vi "OPTICAL BEACON TRACKER.vi"() -> ()   [LabVIEW 2015]
uses:
  <vilib>/userdefined/High Color/IMAQdx.ctl
  <vilib>/vision/driver/NI_Vision_Acquisition_Software.lvlib
  <resource>/objmgr/imaqdx.rc
panel:
  out "Numeric":dbl
  out "Compared":sgl
  out "Optical Beacon Aligned":bool
  in  "Threshhold x":dbl format="%#_13g"
  in  "stop":bool
  out "GREEN X":sgl
  out "RED X":sgl
  in  "Camera":T1
  in  "Stop 3":bool
  out "VA RED IMAGE":T2(plugin-control)
  out "FEED RED":T2(plugin-control)
  out "Processed Image RED":T2(plugin-control)
  out "Video Modes":string
  in  "Video Mode":dbl min=0.0 max=5.0 step=1.0
  out "Y Resoloution":i32
  out "X Resoloution":i32
  in  "Stop 2":bool
  out "VA GREEN Image":T2(plugin-control)
  out "FEED GREEN":T2(plugin-control)
  out "Process Image GREEN":T2(plugin-control)
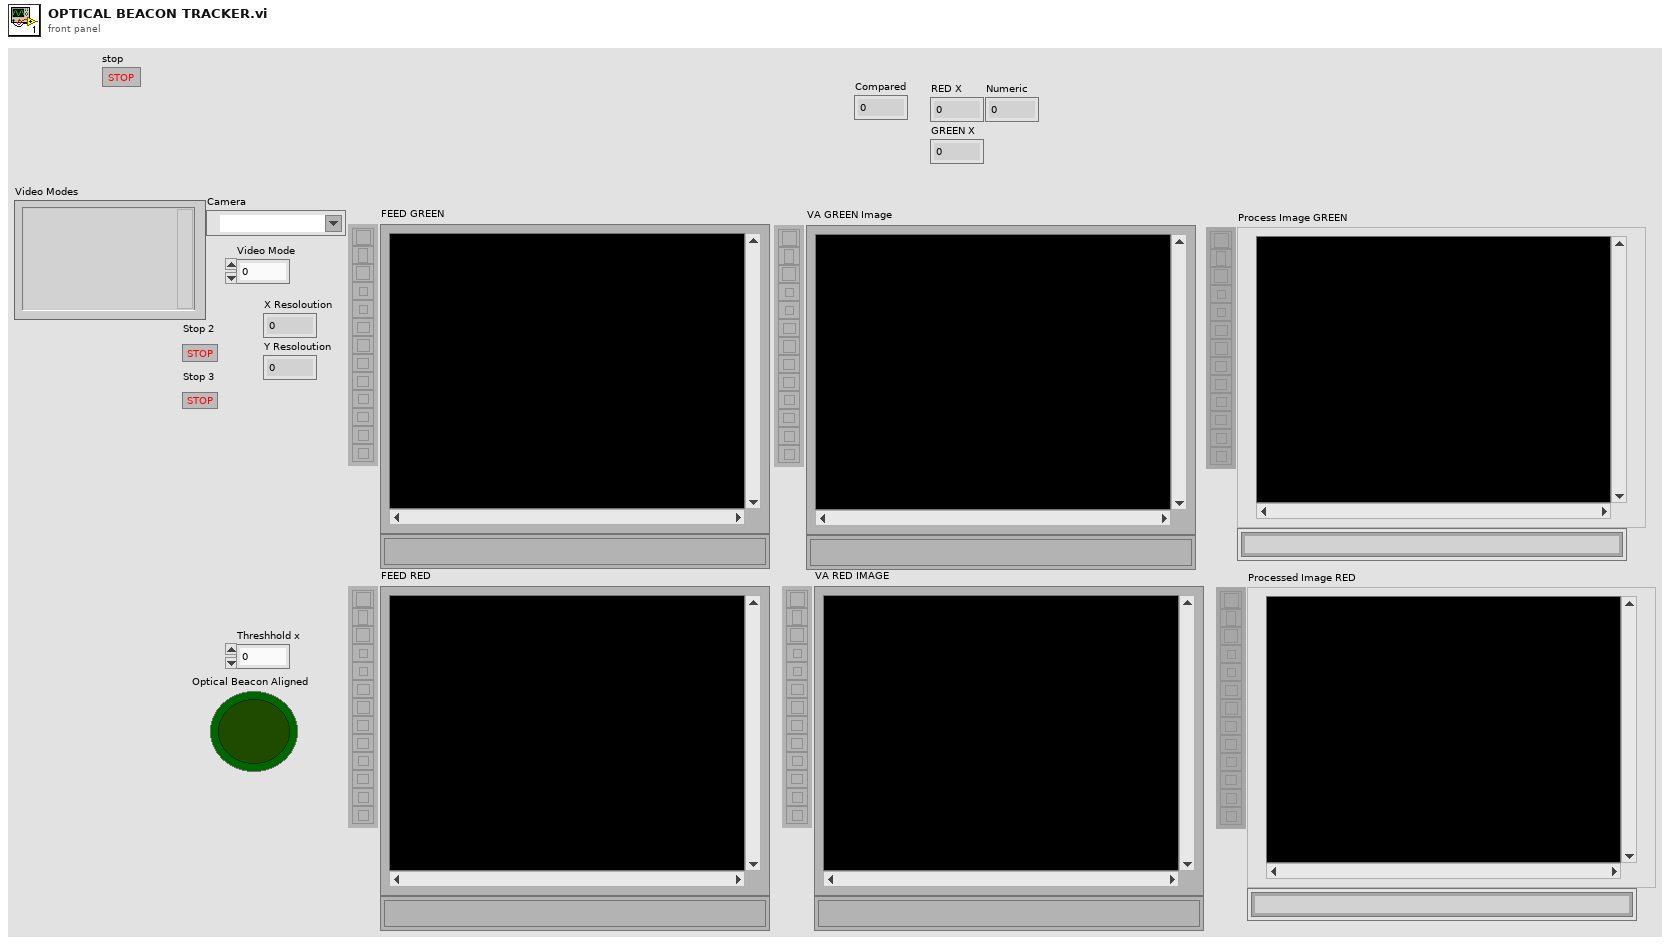
[diagram p1: front panel]
types:
  T1 = typedef "IMAQdx.ctl" = refnum<k21>
  T2 = typedef "IMAQ Image.ctl" = refnum<image>
  T3 = typedef "IMAQ Circle" = cluster{"Center X":i32, "Center Y":i32, "Inner Radius":i32, "Outer Radius":i32, "Start Angle":dbl, "End Angle":dbl}
  T4 = cluster{"Center":cluster{"X":sgl, "Y":sgl}, "Radius":dbl}
  T5 = typedef "ROI Descriptor" = cluster{"Global Rectangle":i32[], "Contours":cluster{"ID":enum32{"External", "Internal"}, "Type":u32, "Coordinates":i32[]}[]}
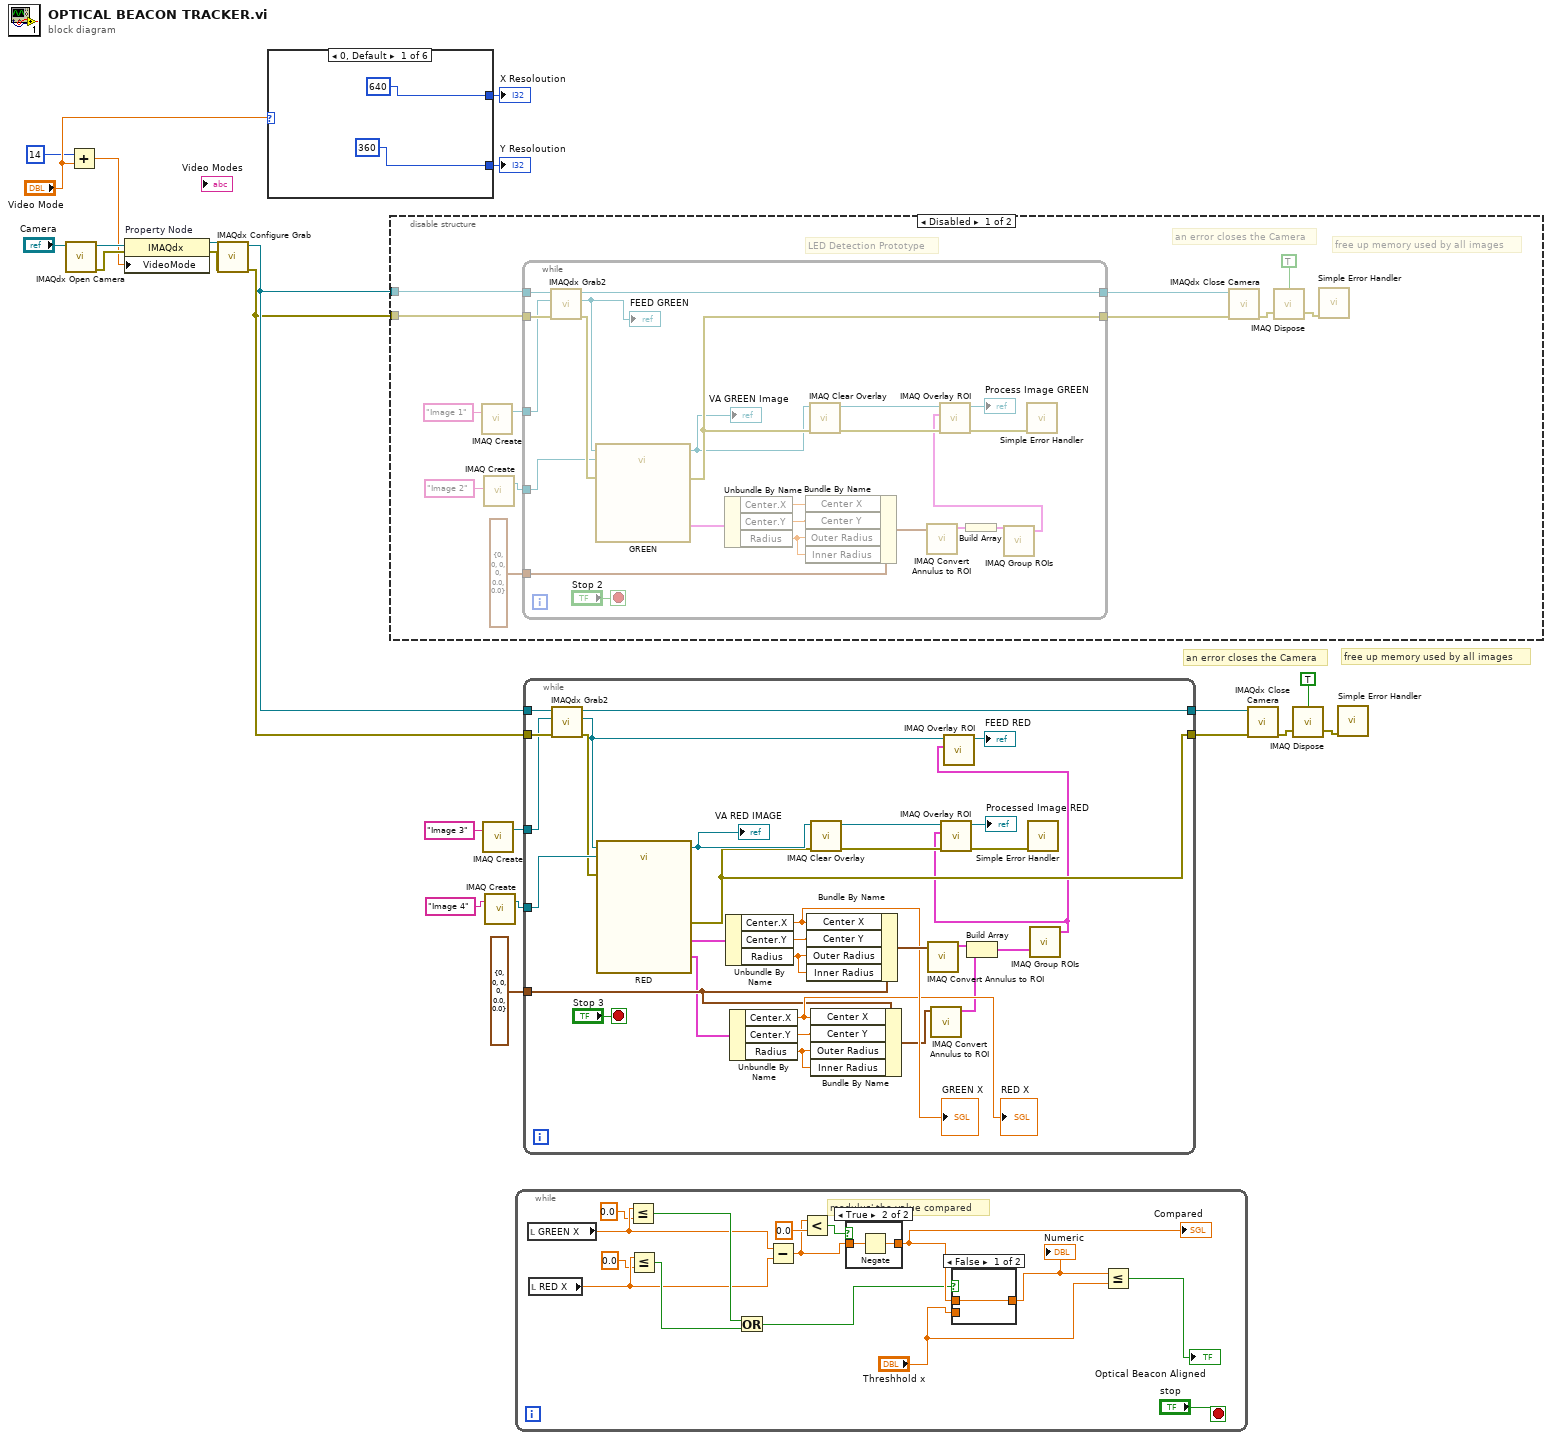
[diagram p0: block diagram]
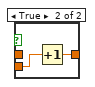
[diagram p2: hidden frame]
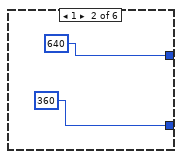
[diagram p5: hidden frame]
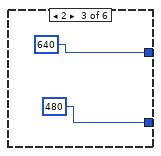
[diagram p6: hidden frame]
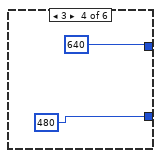
[diagram p7: hidden frame]
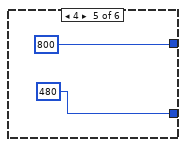
[diagram p8: hidden frame]
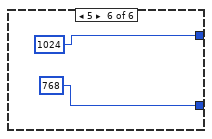
[diagram p9: hidden frame]
diagram:
  # "an error closes the Camera"
  # "free up memory used by all images"
  n1 = call <vilib>:"IMAQdx Open Camera.vi"("Session In"="Camera") -> ("error out"=w21:errorcluster, "Session Out"=w22:T1)  [unwired: 9 in]
  n2 = Add(x=14, y="Video Mode") -> (x+y=w18:dbl)
  n3 = property on="Property Node" class="IMAQdx"(reference=w22, error in=w21, "VideoMode"=w18) -> (reference out=w20:T1, error out=w19:errorcluster)
  n4 = call <vilib>:"IMAQdx Configure Grab.vi"("error in"=w19, "Session In"=w20) -> ("error out"=w4:errorcluster, "Session Out"=w5:T1)  [unwired: 8 in]
  n5 = case shown="0, Default" "Video Mode" {
    tunnel: [640 640 640 640 800 1024] -> w15
    tunnel: [360 360 480 480 480 768] -> w16
    frame 0, Default {
    }
    frame 1 {
    }
    frame 2 {
    }
    frame 3 {
    }
    frame 4 {
    }
    frame 5 {
    }
  }
  "X Resoloution" <- w15
  "Y Resoloution" <- w16
  n6 = disable-structure shown="Disabled" {
    disable-tunnel: w5 -> [w36 _]
    disable-tunnel: w4 -> [w35 _]
    frame Disabled {
      # "LED Detection Prototype"
      # "an error closes the Camera"
      # "free up memory used by all images"
      n7 = call "IMAQ Create"("Image Name"="Image 1") -> ("New Image"=w40:T2)  [unwired: 4 in, 1 out]
      n8 = call "IMAQ Create"("Image Name"="Image 2") -> ("New Image"=w43:T2)  [unwired: 4 in, 1 out]
      n9 = while {
        tunnel: [w51] -> w39
        tunnel: w43 -> [w47]
        tunnel: w35 -> [w69]
        tunnel: w36 -> [w68]
        tunnel: w40 -> [w67]
        tunnel: [w66] -> w38
        tunnel: T3 {"Center X"=0, "Center Y"=0, "Inner Radius"=0, "Outer Radius"=0, "Start Angle"=0.0, "End Angle"=0.0} ("Annulus") -> [w56]
        stop <- "Stop 2" stop-if-true
        n10 = call <vilib>:"IMAQdx Grab2.vi"("error in"=w69, "Image In"=w67, "Session In"=w68) -> ("error out"=w64:errorcluster, "Image Out"=w63:T2, "Session Out"=w66:T1)  [unwired: 5 in, 1 out]
        "FEED GREEN" <- w63
        n11 = call "GREEN"("Image In"=w63, "Image Dst"=w47, "error in"=w64) -> ("Image Out"=w49:T2, "Best Circle (Fit Circle Ball 1)"=w58:T4, "error out"=w51:errorcluster)  [unwired: 1 in, 21 out]
        "VA GREEN Image" <- w49
        n12 = Unbundle By Name(w58) -> ("Center.X"=w50:sgl, "Center.Y"=w59:sgl, "Radius"=w62:dbl)
        n13 = Bundle By Name(cluster=w56, "Center X"=w50, "Center Y"=w59, "Outer Radius"=w62, "Inner Radius"=w62) -> (w57:T3)
        n14 = call "IMAQ Clear Overlay"("error in (no error)"=w51, "Image"=w49) -> ("error out"=w54:errorcluster, "Image Out"=w53:T2)  [unwired: 1 in, 7 out]
        n15 = call "IMAQ Convert Annulus to ROI"("Annulus"=w57) -> ("ROI Descriptor"=w60:T5)  [unwired: 1 in, 8 out]
        n16 = Build Array(w60) -> (w61:T5[])
        n17 = call "IMAQ Group ROIs"("ROI Descriptors"=w61) -> ("ROI Descriptor out"=w52:T5)  [unwired: 1 in, 3 out]
        n18 = call "IMAQ Overlay ROI"("error in (no error)"=w54, "ROI Descriptor"=w52, "Image"=w53) -> ("error out"=w55:errorcluster, "Image Out"=→"Process Image GREEN":T2)  [unwired: 3 in, 4 out]
        n19 = call <vilib>:"Simple Error Handler.vi"("error in (no error)"=w55) -> ()  [unwired: 1 in, 8 out]
      }
      n20 = call <vilib>:"IMAQdx Close Camera.vi"("error in"=w39, "Session In"=w38) -> ("error out"=w44:errorcluster)  [unwired: 9 in]
      n21 = call "IMAQ Dispose"("All Images? (No)"=TRUE, "error in (no error)"=w44) -> ("error out"=w45:errorcluster)  [unwired: 4 in]
      n22 = call <vilib>:"Simple Error Handler.vi"("error in (no error)"=w45) -> ()  [unwired: 4 in, 5 out]
    }
    frame Enabled {
    }
  }
  n23 = call "IMAQ Create"("Image Name"="Image 3") -> ("New Image"=w10:T2)  [unwired: 4 in, 1 out]
  n24 = call "IMAQ Create"("Image Name"="Image 4") -> ("New Image"=w9:T2)  [unwired: 4 in, 1 out]
  n25 = while {
    stop <- "stop" stop-if-true
    # "modulus' the value compared"
    n26 = local read "GREEN X"() -> (w73:sgl)
    n27 = local read "RED X"() -> (w71:sgl)
    n28 = Less Or Equal?(x=w73, y=sgl 0.0) -> (x <= y?=w79:bool)
    n29 = Less Or Equal?(x=w71, y=sgl 0.0) -> (x <= y?=w80:bool)
    n30 = Or(x=w79, y=w80) -> (x .or. y?=w75:bool)
    n31 = Subtract(x=w73, y=w71) -> (x-y=w82:sgl)
    n32 = Less?(x=w82, y=sgl 0.0) -> (x < y?=w81:bool)
    n33 = case shown="True" w81 {
      tunnel: w82 -> [w88 w90]
      tunnel: [w88 w89] -> w76
      frame False {
      }
      frame True {
        n34 = Negate(x=w90) -> (-x=w89:sgl)
      }
    }
    "Compared" <- w76
    n35 = case shown="False" w75 {
      tunnel: "Threshhold x" -> [_ w86]
      tunnel: [w85 w87] -> w77
      tunnel: w76 -> [w85 _]
      frame False {
      }
      frame True {
        n36 = Increment(x=w86) -> (x+1=w87:dbl)
      }
    }
    "Numeric" <- w77
    n37 = Less Or Equal?(x=w77, y="Threshhold x") -> (x <= y?=→"Optical Beacon Aligned":bool)
  }
  n38 = while {
    tunnel: [w101] -> w11
    tunnel: w9 -> [w103]
    tunnel: w4 -> [w120]
    tunnel: w5 -> [w119]
    tunnel: w10 -> [w118]
    tunnel: [w117] -> w12
    tunnel: T3 {"Center X"=0, "Center Y"=0, "Inner Radius"=0, "Outer Radius"=0, "Start Angle"=0.0, "End Angle"=0.0} ("Annulus") -> [w97]
    stop <- "Stop 3" stop-if-true
    n39 = call <vilib>:"IMAQdx Grab2.vi"("error in"=w120, "Image In"=w118, "Session In"=w119) -> ("error out"=w102:errorcluster, "Image Out"=w93:T2, "Session Out"=w117:T1)  [unwired: 5 in, 1 out]
    n40 = call "RED"("Image In"=w93, "Image Dst"=w103, "error in"=w102) -> ("Image Out"=w105:T2, "Best Circle (Fit Circle Ball 1)"=w111:T4, "error out"=w101:errorcluster, "Best Circle (Fit Circle Ball 2)"=w91:T4)  [unwired: 2 in, 19 out]
    "VA RED IMAGE" <- w105
    n41 = Unbundle By Name(w111) -> ("Center.X"=w106:sgl, "Center.Y"=w112:sgl, "Radius"=w115:dbl)
    "GREEN X" <- w106
    n42 = Unbundle By Name(w91) -> ("Center.X"=w100:sgl, "Center.Y"=w99:sgl, "Radius"=w98:dbl)
    "RED X" <- w100
    n43 = Bundle By Name(cluster=w97, "Center X"=w106, "Center Y"=w112, "Outer Radius"=w115, "Inner Radius"=w115) -> (w110:T3)
    n44 = call "IMAQ Clear Overlay"("error in (no error)"=w101, "Image"=w105) -> ("error out"=w108:errorcluster, "Image Out"=w107:T2)  [unwired: 1 in, 7 out]
    n45 = Bundle By Name(cluster=w97, "Center X"=w100, "Center Y"=w99, "Outer Radius"=w98, "Inner Radius"=w98) -> (w96:T3)
    n46 = call "IMAQ Convert Annulus to ROI"("Annulus"=w110) -> ("ROI Descriptor"=w113:T5)  [unwired: 1 in, 8 out]
    n47 = call "IMAQ Convert Annulus to ROI"("Annulus"=w96) -> ("ROI Descriptor"=w95:T5)  [unwired: 1 in, 8 out]
    n48 = Build Array(w113, w95) -> (w114:T5[])
    n49 = call "IMAQ Group ROIs"("ROI Descriptors"=w114) -> ("ROI Descriptor out"=w92:T5)  [unwired: 1 in, 3 out]
    n50 = call "IMAQ Overlay ROI"("error in (no error)"=w108, "ROI Descriptor"=w92, "Image"=w107) -> ("error out"=w109:errorcluster, "Image Out"=→"Processed Image RED":T2)  [unwired: 3 in, 4 out]
    n51 = call "IMAQ Overlay ROI"("ROI Descriptor"=w92, "Image"=w93) -> ("Image Out"=→"FEED RED":T2)  [unwired: 4 in, 5 out]
    n52 = call <vilib>:"Simple Error Handler.vi"("error in (no error)"=w109) -> ()  [unwired: 1 in, 8 out]
  }
  n53 = call <vilib>:"IMAQdx Close Camera.vi"("error in"=w11, "Session In"=w12) -> ("error out"=w8:errorcluster)  [unwired: 9 in]
  n54 = call "IMAQ Dispose"("All Images? (No)"=TRUE, "error in (no error)"=w8) -> ("error out"=w7:errorcluster)  [unwired: 4 in]
  n55 = call <vilib>:"Simple Error Handler.vi"("error in (no error)"=w7) -> ()  [unwired: 4 in, 5 out]
